vi "PreConfigured Instruments.vi"() -> (3 "PreConfigured Instruments":T1[](array[typedef]) {"Private"."Offset" format="%^_3e"; "Private"."Scale Factors" format="%^_3e"})   [LabVIEW 2024]
doc: "Regularize paths to preconfigured instruments for cross platform compatibility"
uses:
  Sub Controls/Instrument Properties.ctl
  Sub Controls/Public.ctl
  Sub Controls/Private.ctl
  Sub Controls/Instrument Ref.ctl
  Sub Controls/SystemCheckBox-resize.ctl
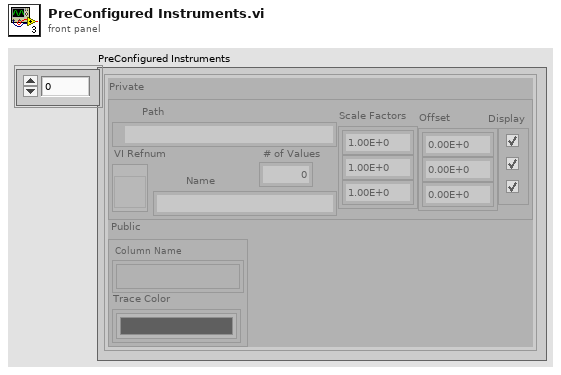
[diagram p1: front panel]
types:
  T1 = typedef "Instrument Properties.ctl" = cluster{"Public":T2, "Private":T3}
  T2 = typedef "Public.ctl" = cluster{"Column Name":string[], "Trace Color":u32[]}
  T3 = typedef "Private.ctl" = cluster{"Path":path, "VI Refnum":T4, "Name":string, "# of Values":i32, "Scale Factors":dbl[], "Display":T5[], "Offset":dbl[]}
  T4 = typedef "Instrument Ref.ctl" = refnum<vi>
  T5 = typedef "SystemCheckBox-resize.ctl" = bool
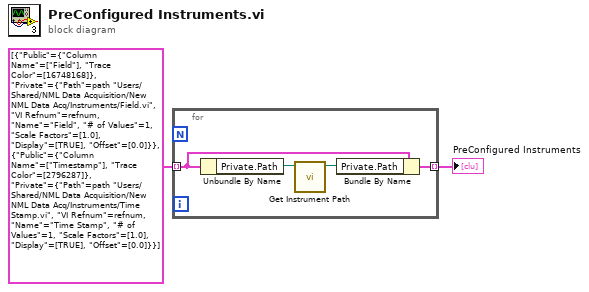
[diagram p0: block diagram]
diagram:
  n1 = for {
    tunnel: T1[] [{"Public"={"Column Name"=["Field"], "Trace Color"=[16748168]}, "Private"={"Path"=path "/Users/Shared/NML Data Acquisition/New NML Data Acq/Instruments/Field.vi", "VI Refnum"=refnum, "Name"="Field", "# of Values"=1, "Scale Factors"=[1.0], "Display"=[TRUE], "Offset"=[0.0]}}, {"Public"={"Column Name"=["Timestamp"], "Trace Color"=[2796287]}, "Private"={"Path"=path "/Users/Shared/NML Data Acquisition/New NML Data Acq/Instruments/Time Stamp.vi", "VI Refnum"=refnum, "Name"="Time Stamp", "# of Values"=1, "Scale Factors"=[1.0], "Display"=[TRUE], "Offset"=[0.0]}}] ("Setup") -> [w5] mode=indexing
    tunnel: [w4] -> w2 mode=indexing
    n2 = Unbundle By Name(w5) -> ("Private.Path"=w6:path)
    n3 = call "Get Instrument Path.vi"("VI Name"=w6) -> ("Instrument Path"=w3:path)  [unwired: 9 in, 1 out]
    n4 = Bundle By Name(cluster=w5, "Private.Path"=w3) -> (w4:T1)
  }
  "PreConfigured Instruments" <- w2
